vi "get_x_iteration_values.vi"(8 "error in (no error)":errorcluster, 11 "TrajectoryAK101022Resonance in":refnum<class "TrajectoryAK101022Resonance.lvclass">) -> (0 "error out":errorcluster, 1 "fly-back offset [iterations]":u16, 2 "fly-forward offset [iterations]":u16, 3 "TrajectoryAK101022Resonance out":refnum<class "TrajectoryAK101022Resonance.lvclass">, 4 "iterations per pixel":u16, 5 "scan segment [iterations]":u16)   [LabVIEW 2010, in "TrajectoryAK101022Resonance.lvclass"]
uses:
  TrajectoryAK101022Resonance.lvclass
  FPGAWrapper/FPGAWrapperAK101022Resonance/FPGAWrapperAK101022Resonance/FPGAWrapperAK101022Resonance.lvclass
  TrajectoryAK101022Resonance.lvclass/TrajectoryAK101022Resonance.ctl
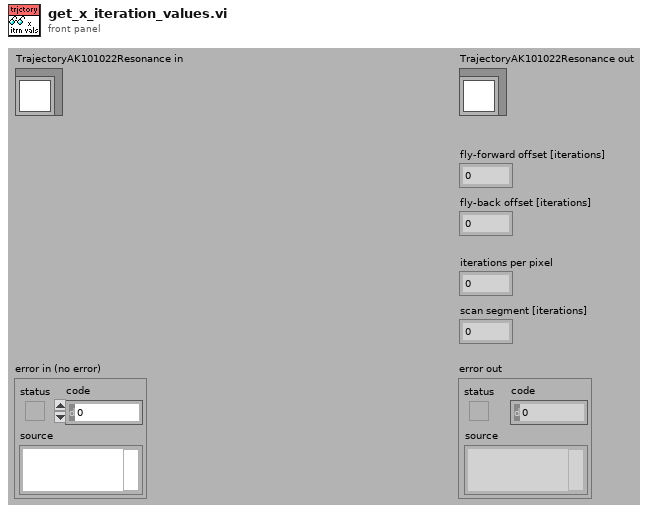
[diagram p1: front panel]
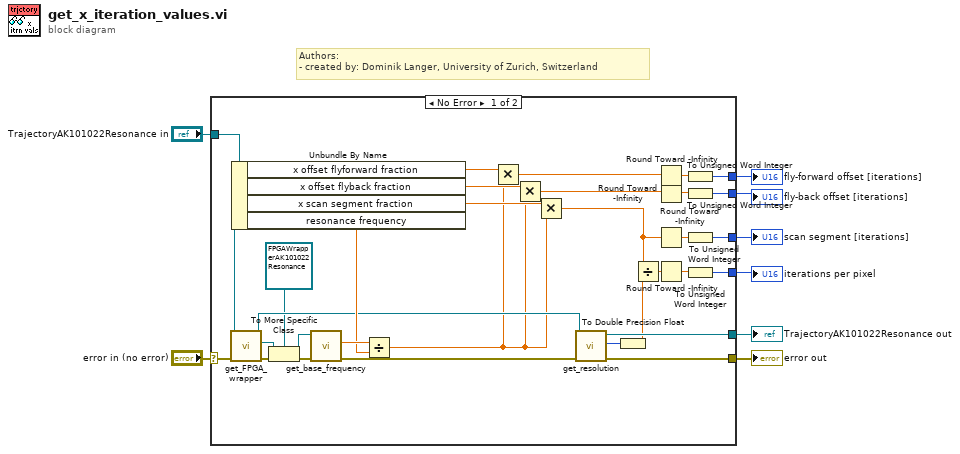
[diagram p0: block diagram]
diagram:
  # "Authors: \n- created by: Dominik Langer, University of Zurich, Switzerland"
  n1 = case shown="No Error" "error in (no error)" {
    selector: "error in (no error)" -> [w39 w41]
    tunnel: [w24 w41] -> w7
    tunnel: [w26 w40] -> w5
    tunnel: "TrajectoryAK101022Resonance in" -> [w20 w40]
    tunnel: [w33 _] -> w4
    tunnel: [w27 _] -> w3
    tunnel: [w14 _] -> w2
    tunnel: [w17 _] -> w1
    frame No Error {
      n2 = call-dynamic "get_FPGA_wrapper.vi"("error in (no error)"=w39, "TrajectoryMG100122GenericFPGA in"=w20) -> ("error out"=w11:errorcluster, "GenericFPGAWrapper.lvclass"=w12:refnum<class "GenericFPGAWrapper.lvclass">, "TrajectoryMG100122GenericFPGA out"=w19:refnum<class "TrajectoryAK101022Resonance.lvclass">)  [unwired: 7 in]
      n3 = Unbundle By Name(w20) -> ("x offset flyforward fraction"=w36:dbl, "x offset flyback fraction"=w32:dbl, "x scan segment fraction"=w31:dbl, "resonance frequency"=w37:dbl[unit])
      n4 = To More Specific Class(target class=refnum<class "FPGAWrapperAK101022Resonance.lvclass"> refnum ("FPGAWrapperAK101022Resonance.lvclass"), reference=w12, error in=w11) -> (specific class reference=w9:refnum<class "FPGAWrapperAK101022Resonance.lvclass">, error out=w10:errorcluster)
      n5 = call "get_base_frequency.vi"("error in (no error)"=w10, "FPGAWrapperAK101022Resonance in"=w9) -> ("error out"=w25:errorcluster, "base frequency"=w38:dbl[unit])  [unwired: 7 in, 1 out]
      n6 = Divide(x=w38, y=w37) -> (x/y=w18:dbl)
      n7 = Multiply(x=w36, y=w18) -> (x*y=w35:dbl)
      n8 = Multiply(x=w32, y=w18) -> (x*y=w28:dbl)
      n9 = Multiply(x=w31, y=w18) -> (x*y=w15:dbl)
      n10 = call-dynamic "get_resolution.vi"("error in (no error)"=w25, "TrajectoryAK101022Resonance in"=w19) -> ("error out"=w24:errorcluster, "x resolution"=w23:i32, "TrajectoryAK101022Resonance out"=w26:refnum<class "TrajectoryAK101022Resonance.lvclass">)  [unwired: 6 in, 1 out]
      n11 = To Double Precision Float(number=w23) -> (double precision float=w22:dbl)
      n12 = Divide(x=w15, y=w22) -> (x/y=w21:dbl)
      n13 = Round Toward -Infinity(1:w35) -> (0:w34:dbl)
      n14 = Round Toward -Infinity(1:w28) -> (0:w30:dbl)
      n15 = Round Toward -Infinity(1:w15) -> (0:w16:dbl)
      n16 = Round Toward -Infinity(1:w21) -> (0:w29:dbl)
      n17 = To Unsigned Word Integer(number=w34) -> (unsigned 16bit integer=w33:u16)
      n18 = To Unsigned Word Integer(number=w30) -> (unsigned 16bit integer=w27:u16)
      n19 = To Unsigned Word Integer(number=w16) -> (unsigned 16bit integer=w17:u16)
      n20 = To Unsigned Word Integer(number=w29) -> (unsigned 16bit integer=w14:u16)
    }
    frame Error {
    }
  }
  "error out" <- w7
  "TrajectoryAK101022Resonance out" <- w5
  "fly-forward offset [iterations]" <- w4
  "fly-back offset [iterations]" <- w3
  "iterations per pixel" <- w2
  "scan segment [iterations]" <- w1
